vi "Interpolate and load IQ samples to memo.vi"(6 "wr.start addr":u32, 7 "burst memo":T1, 9 "wr.enable":bool, 11 "DRAM resources":T2={"DRAM read data FIFO"="", "DRAM write data FIFO"="", "DRAM request FIFO"="", "DRAM U512 memo"=refnum, "DMA data loader"="custom data", "BRAM read data FIFO"="", "BRAM write data FIFO"="", "BRAM request FIFO"="", "BRAM U512 memo"=refnum}) -> ()   [LabVIEW 2019, in "TX burst sequencer.lvlib"]
uses:
  TX burst sequencer.lvlib
  DRAM resources.ctl
  <instrlib>/_niInstr/Memory/v1/FPGA/DRAM U512/niInstr Memory DRAM U512 v1 FPGA.lvclass
  <instrlib>/_niInstr/Memory/v1/FPGA/BRAM U512/niInstr Memory BRAM U512 v1 FPGA.lvclass
  Burst memo.ctl
  <vilib>/rvi/DataTransferAndStorage/Container/Common/niFpgaContainerGetUniqueNameForEmu.vi
  <vilib>/rvi/DataTransferAndStorage/Container/Common/niFpgaContainerSetEmuInfo.vi
  <vilib>/rvi/eio/common/nirviEmuReportErrorAndStop.vi
  <vilib>/rvi/DataTransferAndStorage/Container/Common/niFpgaContainerExecOnDevCompGetState.vi
  <vilib>/rvi/Emulation/niFpgaEmulationIsFPGAContextNoSignature.vi
  <vilib>/rvi/Emulation/niFpgaSctlEmulationGetInTimedLoop.vi
  <vilib>/rvi/errors/niFpgaSetErrorForExecOnDevCompSimple.vi
  <vilib>/rvi/FIFO/Fifo_Resource/nirvififoEmulationSetSize.vi
  <vilib>/rvi/FIFO/Fifo_Resource/nirviFifoEmulationQueueMgr.vi
  <instcachedir>/0/nirviFifoEmulationQueueMgr_E5CAEC123FF24DC58D834DCA3CDAA9B5.lvgen/nirviFifoEmulationQueueMgr_E5CAEC123FF24DC58D834DCA3CDAA9B5_017.vi
  <vilib>/rvi/FIFO/Fifo_Resource/nirvififoEmulationDetermineInputValidOut.vi
  <vilib>/rvi/FIFO/Fifo_Resource/nirvififoEmulationCreateLock.vi
  <vilib>/rvi/Emulation/niFpgaProcessEmulError.vi
  <vilib>/rvi/FIFO/Fifo_Resource/nirvififoEmulationObtainLock.vi
  <vilib>/rvi/FIFO/Fifo_Resource/nirvififoEmulationReleaseLock.vi
  <vilib>/rvi/occurrence/nirviWaitOnOccurrenceBase.vi
  <vilib>/rvi/errors/nirviReportUnexpectedCaseInternalError.vi
  <vilib>/rvi/errors/nirviReportUnexpectedCaseInternalError (U32).vi
  <vilib>/Utility/error.llb/Clear Errors.vi
  <vilib>/rvi/interface/RandomDataEmulation/niFpgaRandomDataHandleErrors.vi
  <vilib>/rvi/interface/RandomDataEmulation/nirviRandomDataAcquireLock.vi
  <vilib>/rvi/interface/RandomDataEmulation/nirviRandomDataQueueStore.vi
  <vilib>/rvi/interface/RandomDataEmulation/nirviRandomDataReleaseLock.vi
  <vilib>/rvi/interface/RandomDataEmulation/nirviFPGAContextMergeError.vi
  <vilib>/rvi/interface/RandomDataEmulation/nirviRandomDataCheckExitLoopConditions.vi
  <vilib>/express/rvi/timingcommon/nirviCommon.vi
  <instrlib>/_niInstr/Data Formatting/v1/FPGA/Private/Convert/FXP(+-,14,1) array to Boolean Array.vi
  <vilib>/rvi/LocalResourceManager/LocalResourceManager.xnode
  <vilib>/rvi/DataTransferAndStorage/Container/XNode/niFpgaContainer.xnode
  <vilib>/rvi/FIFO/Fifo_Resource/niFpgaFifoEmulationRefIn.vi
  <vilib>/rvi/FIFO/Fifo_Resource/niFpgaFifoEmulationRefInMultiElement.vi
  <instrlib>/_niInstr/Basic Elements/v1/FPGA/niInstr Basic Elements v1 FPGA.lvlib
  Utility/FPGA Utility.lvlib
  <instrlib>/_niInstr/Data Formatting/v1/FPGA/niInstr Data Formatting v1 FPGA.lvlib
panel:
  out "samples interpolated":u32
  out "input consumed":bool[](array[boolean])
  in  "burst size":u32
  in  "input sample rate":fxp<+,48,1>
  in  "clock x 2":refnum<k21>
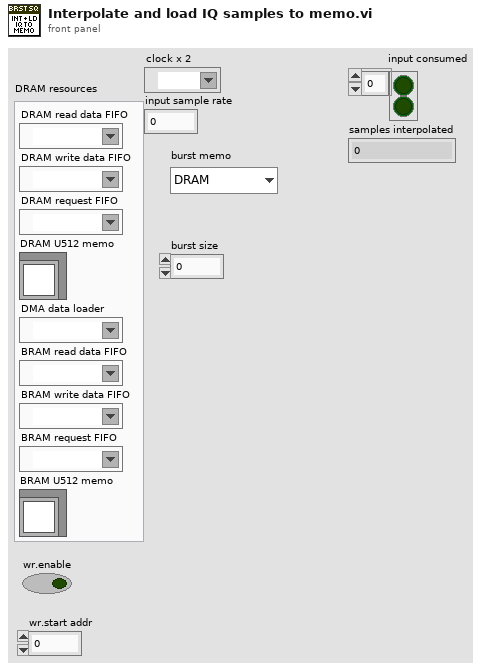
[diagram p1: front panel]
types:
  T1 = typedef "TX burst sequencer.lvlib/Burst memo.ctl" = enum16{"DRAM", "BRAM"}
  T2 = typedef "TX burst sequencer.lvlib/DRAM resources.ctl" = cluster{"DRAM read data FIFO":refnum<k21>, "DRAM write data FIFO":refnum<k21>, "DRAM request FIFO":refnum<k21>, "DRAM U512 memo":refnum<class "niInstr Memory DRAM U512 v1 FPGA.lvclass">, "DMA data loader":refnum<k21>, "BRAM read data FIFO":refnum<k21>, "BRAM write data FIFO":refnum<k21>, "BRAM request FIFO":refnum<k21>, "BRAM U512 memo":refnum<class "niInstr Memory BRAM U512 v1 FPGA.lvclass">}
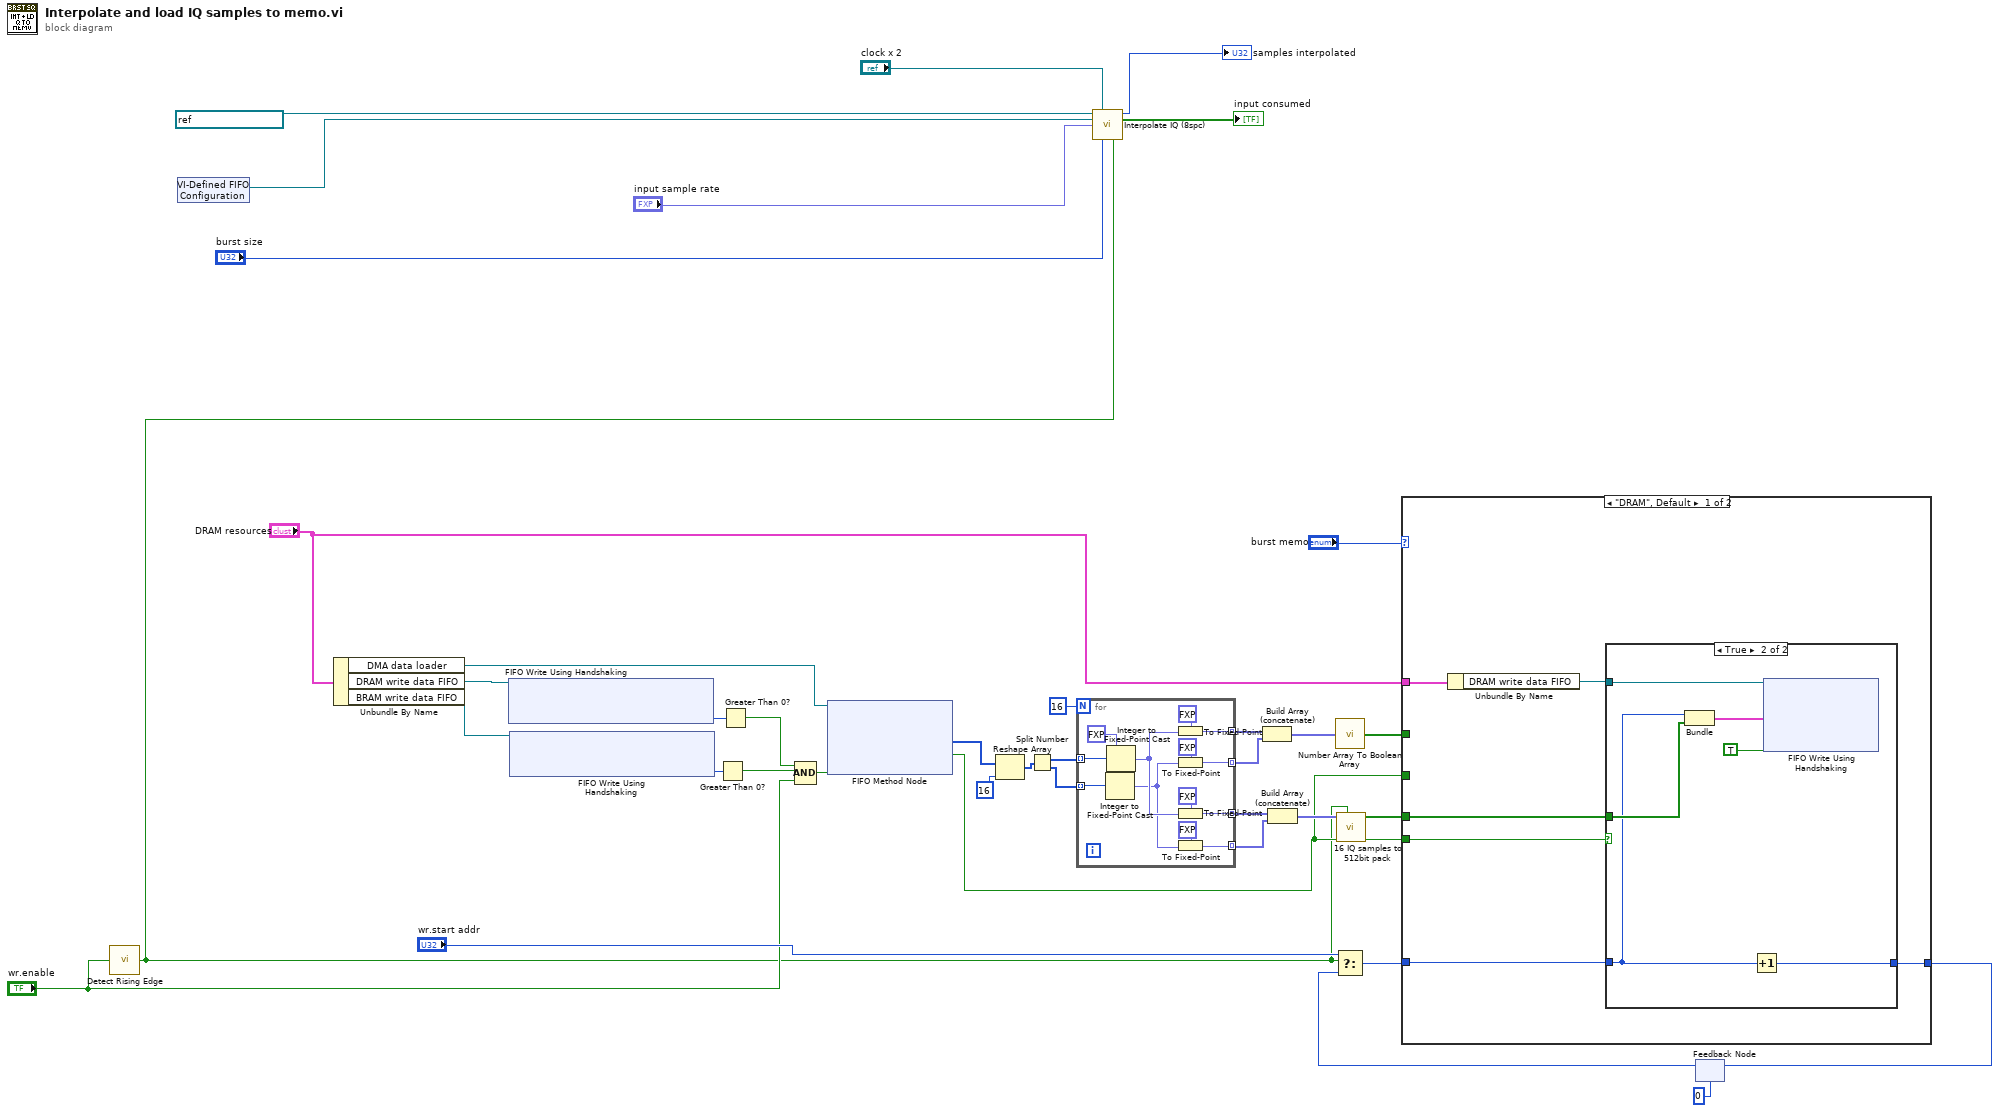
[diagram p0: block diagram]
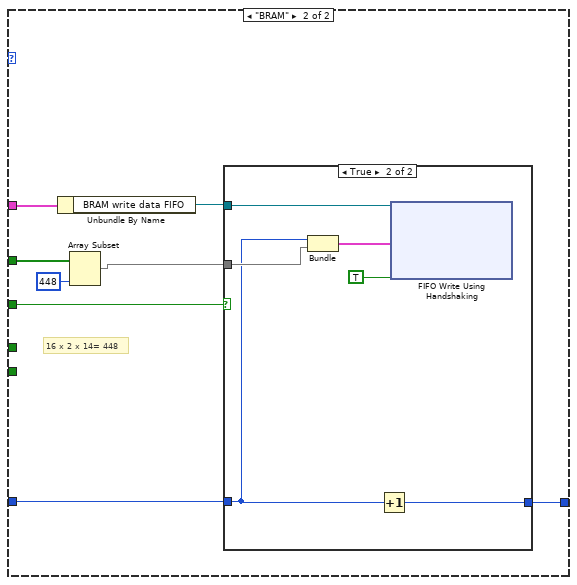
[diagram p3: hidden frame]
diagram:
  n1 = call <instrlib>:"Detect Rising Edge.vi"("signal"="wr.enable") -> ("edge detected"=w1:bool)  [unwired: 14 in]
  n2 = xnode "VI-Defined FIFO Configuration"() -> ("FIFO Out"=w6:refnum<k21>)
  n3 = Unbundle By Name("DRAM resources") -> ("DMA data loader"=w31:refnum<k21>, "DRAM write data FIFO"=w32:refnum<k21>, "BRAM write data FIFO"=w17:refnum<k21>)
  n4 = xnode ("FIFO Write Using Handshaking")("FIFO In"=w32) -> ("Number of Elements to Write"=w38:u32)  [unwired: 1 out]
  n5 = xnode ("FIFO Write Using Handshaking")("FIFO In"=w17) -> ("Number of Elements to Write"=w16:u32)  [unwired: 1 out]
  n6 = Greater Than 0?(x=w16) -> (x > 0?=w15:bool)
  n7 = Greater Than 0?(x=w38) -> (x > 0?=w40:bool)
  n8 = Compound Arithmetic op=AND(w40, w15, "wr.enable") -> (w39:bool)
  n9 = xnode ("FIFO Method Node")("Ready for Output"=w39, "FIFO In"=w31) -> ("Element"=w26:u32[], "Output Valid"=w11:bool)  [unwired: 1 out]
  n10 = Reshape Array(w26, 16 ("dimension size")) -> (w29:u32[])
  n11 = Split Number(x=w29) -> (hi(x)=w28:u16[], lo(x)=w27:u16[])
  n12 = for {
    N: 16 -> [_]
    tunnel: w28 -> [w53] mode=indexing
    tunnel: w27 -> [w52] mode=indexing
    tunnel: [w48] -> w24 mode=indexing
    tunnel: [w47] -> w23 mode=indexing
    tunnel: [w42] -> w19 mode=indexing
    tunnel: [w41] -> w20 mode=indexing
    w51 = fxp<+/-,16,1> 0.0 ("fixed-point type")
    n13 = Integer to Fixed-Point Cast(fixed-point type=w51, integer=w52) -> (fixed-point=w43:fxp<+/-,16,1>)
    n14 = Integer to Fixed-Point Cast(fixed-point type=w51, integer=w53) -> (fixed-point=w46:fxp<+/-,16,1>)
    n15 = To Fixed-Point(fixed-point type=fxp<+/-,14,1> 0.0, number=w46) -> (fixed-point=w41:fxp<+/-,14,1>)
    n16 = To Fixed-Point(fixed-point type=fxp<+/-,14,1> 0.0, number=w43) -> (fixed-point=w42:fxp<+/-,14,1>)
    n17 = To Fixed-Point(fixed-point type=fxp<+/-,12,1> 0.0, number=w46) -> (fixed-point=w48:fxp<+/-,12,1>)
    n18 = To Fixed-Point(fixed-point type=fxp<+/-,12,1> 0.0, number=w43) -> (fixed-point=w47:fxp<+/-,12,1>)
  }
  n19 = call "Interpolate IQ (8spc).vi"("data in FIFO"=refnum<k21> "data loader 8spc" ("FIFO In"), "Clock x2"="clock x 2", "data out FIFO - interpolated"=w6, "input sample rate"="input sample rate", "burst size"="burst size", "reset"=w1) -> ("count out"=→"samples interpolated":u32, "input consumed"=→"input consumed":bool[])  [unwired: 8 in]
  n20 = Build Array (concatenate)(w20, w19) -> (w18:fxp<+/-,14,1>[])
  n21 = Build Array (concatenate)(w24, w23) -> (w22:fxp<+/-,12,1>[])
  n22 = call-poly <instrlib>:"Number Array To Boolean Array.vi"("data in"=w18) -> ("data out"=w12:bool[])  [unwired: 14 in]
  n23 = call "16 IQ samples to 512bit pack.vi"("reset"=w1, "input valid"=w11, "data in"=w22) -> ("output valid"=w21:bool, "data out"=w10:bool[])  [unwired: 6 in, 1 out]
  n24 = feedback #1(u32 0) -> (w36:u32)
  n25 = Select(t="wr.start addr", s=w1, f=w36) -> (s? t:f=w34:u32)
  n26 = case shown="\"DRAM\", Default" "burst memo" {
    tunnel: [w59 w74] -> w35
    tunnel: w34 -> [w58 w73]
    tunnel: w21 -> [w57 _]
    tunnel: "DRAM resources" -> [w56 w72]
    tunnel: w12 -> [_ w69]
    tunnel: w11 -> [_ w70]
    tunnel: w10 -> [w54 _]
    frame "DRAM", Default {
      n27 = Unbundle By Name(w56) -> ("DRAM write data FIFO"=w55:refnum<k21>)
      n28 = case shown="True" w57 {
        tunnel: w54 -> [_ w65]
        tunnel: w55 -> [_ w66]
        tunnel: w58 -> [w60 w62]
        tunnel: [w60 w61] -> w59
        frame False {
        }
        frame True {
          n29 = Bundle("wr.start addr"=w62, "data out"=w65) -> (w64:cluster{"wr.start addr":u32, "data out":bool[]})  [unwired: 1 in]
          n30 = Increment(x=w62) -> (x+1=w61:u32)
          n31 = xnode ("FIFO Write Using Handshaking")("Element"=w64, "Input Valid"=TRUE, "FIFO In"=w66) -> ()  [unwired: 2 out]
        }
      }
    }
    frame "BRAM" {
      # "16 x 2 x 14= 448"
      n32 = Unbundle By Name(w72) -> ("BRAM write data FIFO"=w71:refnum<k21>)
      n33 = Array Subset(array=w69, length=448) -> (w67:bool[])  [unwired: 1 in]
      n34 = case shown="True" w70 {
        tunnel: w67 -> [_ w80]
        tunnel: w71 -> [_ w81]
        tunnel: w73 -> [w75 w77]
        tunnel: [w75 w76] -> w74
        frame False {
        }
        frame True {
          n35 = Bundle("wr.start addr"=w77, w80) -> (w79:cluster{"wr.start addr":u32, bool[]})  [unwired: 1 in]
          n36 = Increment(x=w77) -> (x+1=w76:u32)
          n37 = xnode ("FIFO Write Using Handshaking")("Element"=w79, "Input Valid"=TRUE, "FIFO In"=w81) -> ()  [unwired: 2 out]
        }
      }
    }
  }
  n38 = feedback-in #1(w35) -> ()
